vi "autonSample.vi"(0 "Auton Array":dbl[][](array[numeric]), 5 "MeasuredHeading":dbl, 9 "EncoderDistance":dbl) -> (4 "Left Drive":dbl(knob) scale=-1.0..1.0, 6 "Right Drive":dbl(knob) scale=-1.0..1.0, 10 "Misc1":dbl, 13 "Misc3":dbl, 14 "Misc4":dbl, 15 "Misc2":dbl)   [LabVIEW 2011]
uses:
  Robot Global Data.vi
  <vilib>/addons/control/pid/pid.llb/PID (DBL).vi
  <vilib>/addons/control/pid/NI_PID_pid.lvlib
panel:
  out "ArrayIndex":u16
  out "Tzero":i64
  out "AccumDist":dbl
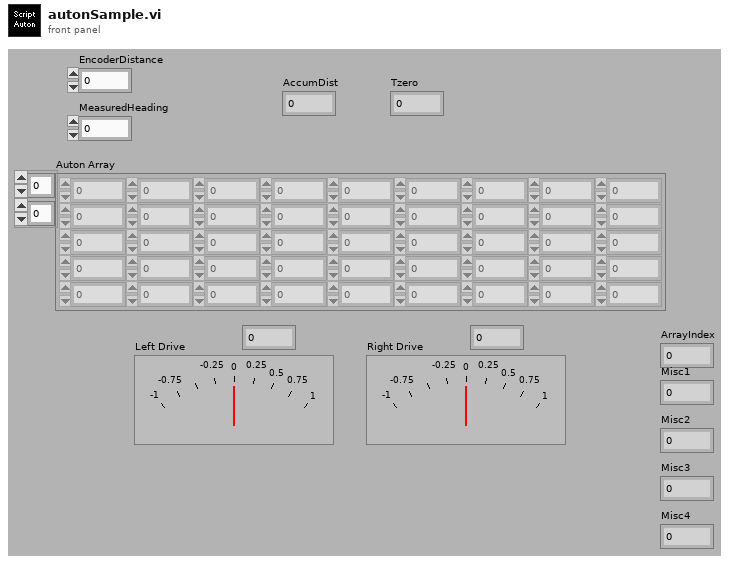
[diagram p1: front panel]
types:
  T1 = cluster{"proportional gain (Kc)":dbl, "integral time (Ti, min)":dbl, "derivative time (Td, min)":dbl}
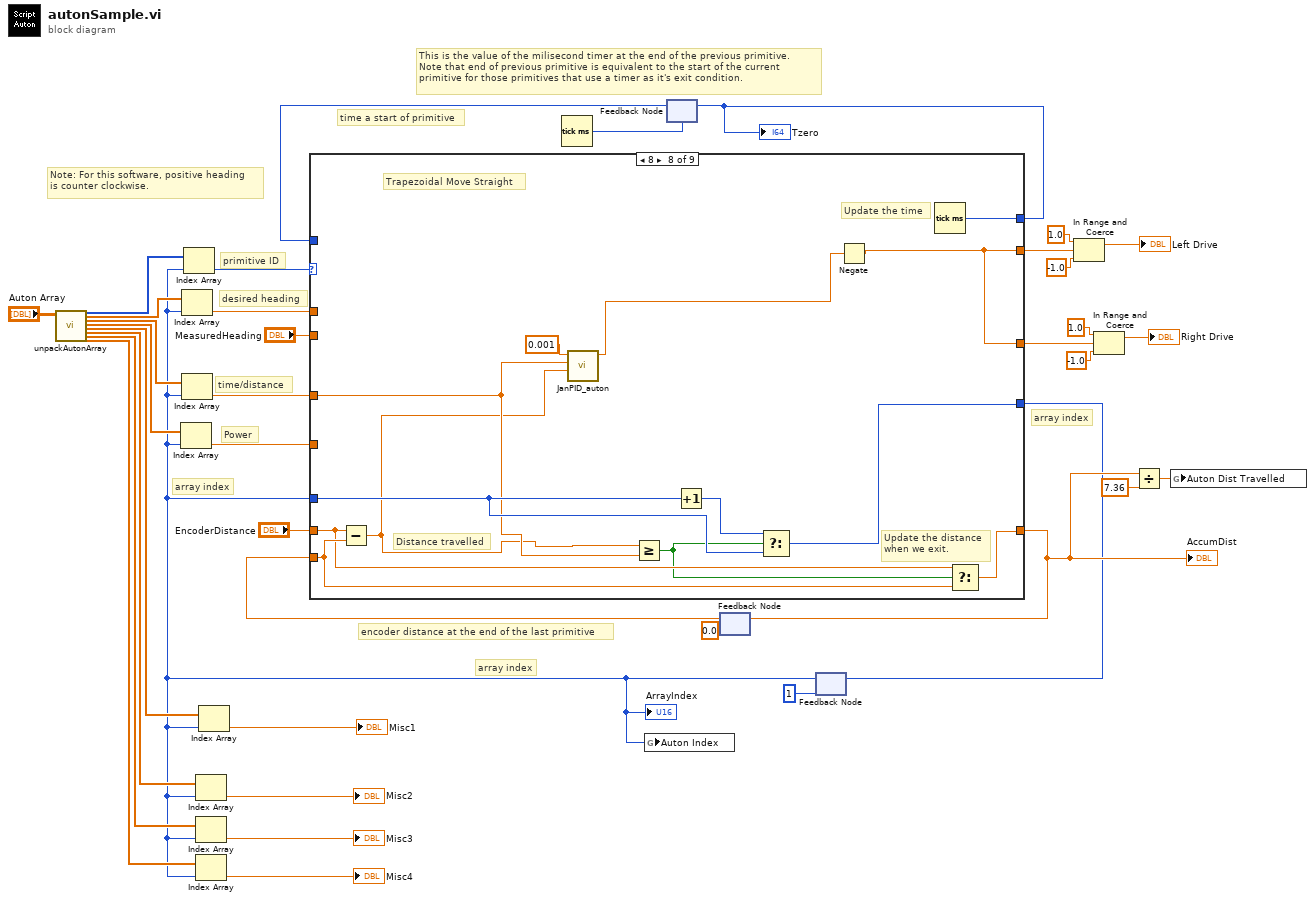
[diagram p0: block diagram]
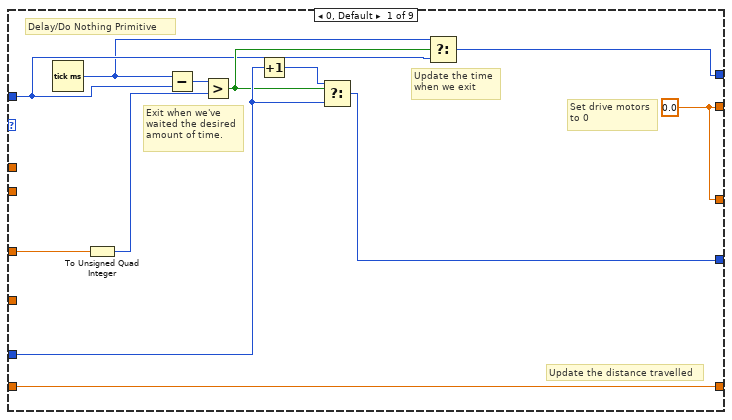
[diagram p2: hidden frame]
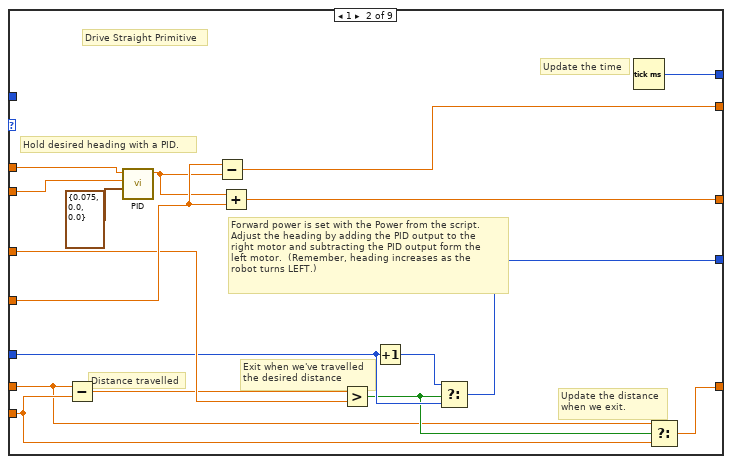
[diagram p3: hidden frame]
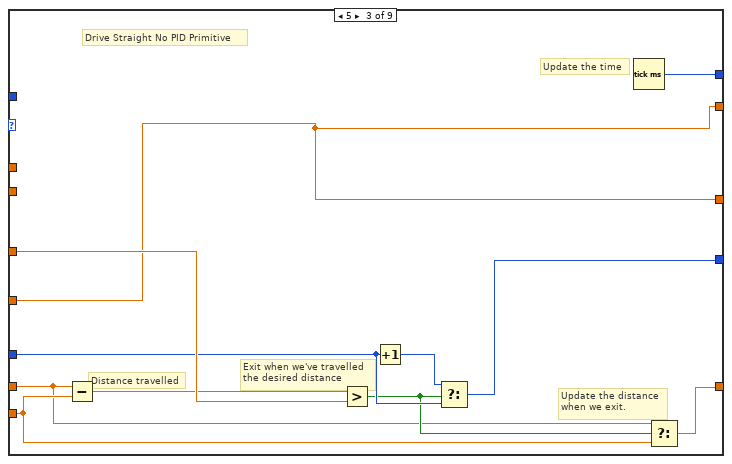
[diagram p4: hidden frame]
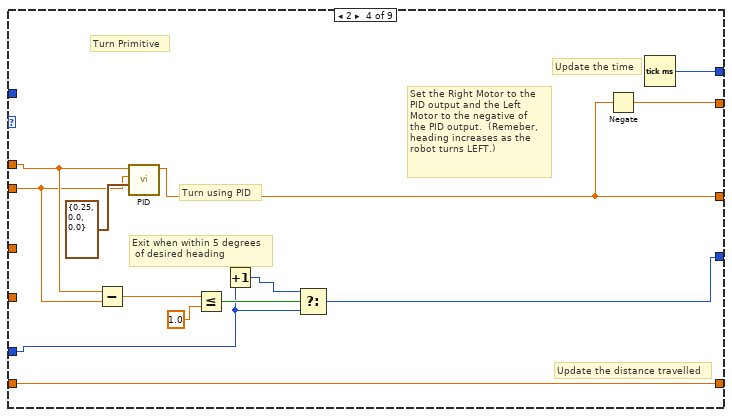
[diagram p5: hidden frame]
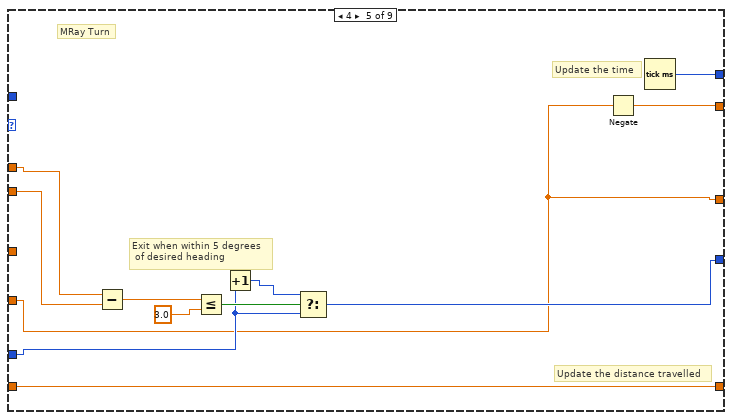
[diagram p6: hidden frame]
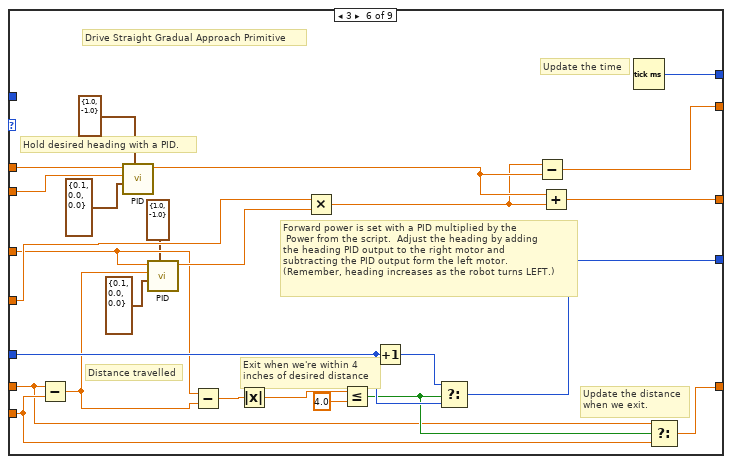
[diagram p7: hidden frame]
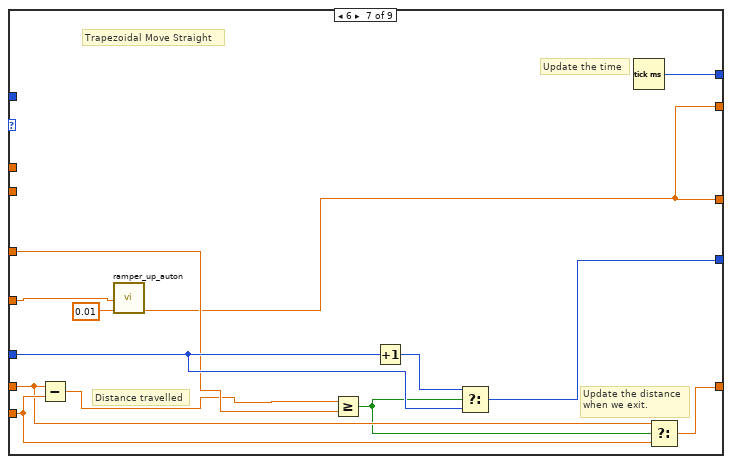
[diagram p8: hidden frame]
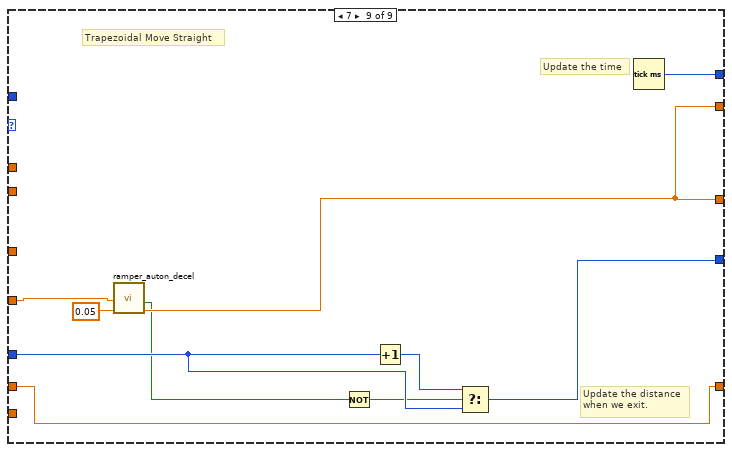
[diagram p9: hidden frame]
diagram:
  # "encoder distance at the end of the last primitive"
  # "Note: For this software, positive heading\nis counter clockwise."
  # "time a start of primitive"
  # "array index"
  # "array index"
  # "This is the value of the milisecond timer at the end of the previous primitive.\nNote that end of previous primitive is equivalent to the start of the current\nprimitive for those primitives that use a timer as it's exit condition."
  # "Power"
  # "array index"
  # "desired heading"
  # "primitive ID"
  # "time/distance"
  n1 = call "unpackAutonArray.vi"("all rows"="Auton Array") -> ("Primitive"=w37:i16[], "Heading"=w19:dbl[], "Distance/Time"=w20:dbl[], "Power"=w17:dbl[], "Misc 1"=w13:dbl[], "Misc 2"=w8:dbl[], "Misc 3"=w7:dbl[], "Misc 4"=w6:dbl[])  [unwired: 1 in, 18 out]
  n2 = Tick Count (ms)() -> (millisecond timer value=w31:u32)
  n3 = feedback #1(w31) -> (w35:u32)
  n4 = feedback #2(0.0 ("EncoderDistance")) -> (w16:dbl)
  n5 = feedback #3(1) -> (w1:i32)
  "ArrayIndex" <- w1
  n6 = Index Array(array=w17, index=w1) -> (element=w33:dbl)
  n7 = Index Array(array=w19, index=w1) -> (element=w18:dbl)
  n8 = Index Array(array=w20, index=w1) -> (element=w34:dbl)
  n9 = Index Array(array=w37, index=w1) -> (element=w36:i16)
  n10 = Index Array(array=w8, index=w1) -> (element=→"Misc2":dbl)
  n11 = Index Array(array=w7, index=w1) -> (element=→"Misc3":dbl)
  n12 = Index Array(array=w6, index=w1) -> (element=→"Misc4":dbl)
  n13 = Index Array(array=w13, index=w1) -> (element=→"Misc1":dbl)
  n14 = case shown="8" w36 {
    tunnel: [w45 w57 w75 w82 w96 w121 w139 w152 w162] -> w2
    tunnel: w1 -> [w47 w58 w76 w83 w97 w122 w140 w153 w163]
    tunnel: [w40 w56 w74 w81 w95 w120 w138 w151 w161] -> w21
    tunnel: w35 -> [w42 _ _ _ _ _ _ _ _]
    tunnel: w34 -> [w49 w60 w78 _ _ w110 w134 w146 _]
    tunnel: w18 -> [_ w67 _ w88 w102 w128 _ _ _]
    tunnel: [w44 w62 w68 w90 w103 w125 w130 w143 w158] -> w29
    tunnel: [w44 w61 w68 w89 w93 w124 w130 w143 w158] -> w22
    tunnel: w33 -> [_ w64 w68 _ w93 w112 w131 _ w159]
    tunnel: "EncoderDistance" -> [w39 w51 w69 w80 w94 w115 w135 w148 w157]
    tunnel: "MeasuredHeading" -> [_ w66 _ w87 w101 w127 _ _ _]
    tunnel: [w39 w54 w72 w80 w94 w119 w137 w150 w157] -> w4
    tunnel: w16 -> [_ w53 w71 _ _ w118 w136 w149 _]
    frame 0, Default {
      w44 = 0.0 ("Numeric")
      # "Update the distance travelled"
      # "Update the time\nwhen we exit"
      # "Exit when we've\nwaited the desired\namount of time."
      # "Set drive motors\nto 0"
      # "Delay/Do Nothing Primitive"
      n15 = Tick Count (ms)() -> (millisecond timer value=w41:u32)
      n16 = To Unsigned Quad Integer(1:w49) -> (0:w48:u64)
      n17 = Subtract(x=w41, y=w42) -> (x-y=w50:u32)
      n18 = Greater?(x=w50, y=w48) -> (0:w43:bool)
      n19 = Increment(x=w47) -> (x+1=w46:i32)
      n20 = Select(t=w46, s=w43, f=w47) -> (s? t:f=w45:i32)
      n21 = Select(t=w41, s=w43, f=w42) -> (s? t:f=w40:u32)
    }
    frame 1 {
      # "Update the distance\nwhen we exit."
      # "Distance travelled"
      # "Forward power is set with the Power from the script.\nAdjust the heading by adding the PID output to the\nright motor and subtracting the PID output form the\nleft motor.  (Remember, heading increases as the\nrobot turns LEFT.)"
      # "Hold desired heading with a PID."
      # "Update the time"
      # "Exit when we've travelled\nthe desired distance"
      # "Drive Straight Primitive"
      n22 = Subtract(x=w51, y=w53) -> (x-y=w55:dbl)
      n23 = call-poly <vilib>:"PID.vi"("PID gains"=T1 {"proportional gain (Kc)"=0.075, "integral time (Ti, min)"=0.0, "derivative time (Td, min)"=0.0}, "process variable"=w66, "setpoint"=w67) -> ("output"=w63:dbl)  [unwired: 3 in, 5 out]
      n24 = Subtract(x=w64, y=w63) -> (x-y=w62:dbl)
      n25 = Add(x=w63, y=w64) -> (x+y=w61:dbl)
      n26 = Greater?(x=w55, y=w60) -> (0:w52:bool)
      n27 = Increment(x=w58) -> (x+1=w59:i32)
      n28 = Select(t=w59, s=w52, f=w58) -> (s? t:f=w57:i32)
      n29 = Tick Count (ms)() -> (millisecond timer value=w56:u32)
      n30 = Select(t=w51, s=w52, f=w53) -> (s? t:f=w54:dbl)
    }
    frame 5 {
      # "Update the distance\nwhen we exit."
      # "Distance travelled"
      # "Update the time"
      # "Exit when we've travelled\nthe desired distance"
      # "Drive Straight No PID Primitive"
      n31 = Subtract(x=w69, y=w71) -> (x-y=w73:dbl)
      n32 = Greater?(x=w73, y=w78) -> (0:w70:bool)
      n33 = Increment(x=w76) -> (x+1=w77:i32)
      n34 = Select(t=w77, s=w70, f=w76) -> (s? t:f=w75:i32)
      n35 = Tick Count (ms)() -> (millisecond timer value=w74:u32)
      n36 = Select(t=w69, s=w70, f=w71) -> (s? t:f=w72:dbl)
    }
    frame 2 {
      # "Update the distance travelled"
      # "Set the Right Motor to the\nPID output and the Left\nMotor to the negative of\nthe PID output.  (Remeber,\nheading increases as the\nrobot turns LEFT.)"
      # "Update the time"
      # "Exit when within 5 degrees\n of desired heading"
      # "Turn using PID"
      # "Turn Primitive"
      n37 = Subtract(x=w88, y=w87) -> (x-y=w79:dbl)
      n38 = call-poly <vilib>:"PID.vi"("PID gains"=T1 {"proportional gain (Kc)"=0.25, "integral time (Ti, min)"=0.0, "derivative time (Td, min)"=0.0}, "process variable"=w87, "setpoint"=w88) -> ("output"=w89:dbl)  [unwired: 3 in, 5 out]
      n39 = Less Or Equal?(x=w79, y=1.0) -> (x <= y?=w85:bool)
      n40 = Increment(x=w83) -> (x+1=w84:i32)
      n41 = Select(t=w84, s=w85, f=w83) -> (s? t:f=w82:i32)
      n42 = Negate(x=w89) -> (-x=w90:dbl)
      n43 = Tick Count (ms)() -> (millisecond timer value=w81:u32)
    }
    frame 4 {
      # "MRay Turn"
      # "Update the distance travelled"
      # "Update the time"
      # "Exit when within 5 degrees\n of desired heading"
      n44 = Subtract(x=w102, y=w101) -> (x-y=w92:dbl)
      n45 = Less Or Equal?(x=w92, y=3.0) -> (x <= y?=w99:bool)
      n46 = Increment(x=w97) -> (x+1=w98:i32)
      n47 = Select(t=w98, s=w99, f=w97) -> (s? t:f=w96:i32)
      n48 = Negate(x=w93) -> (-x=w103:dbl)
      n49 = Tick Count (ms)() -> (millisecond timer value=w95:u32)
    }
    frame 3 {
      # "Update the distance\nwhen we exit."
      # "Distance travelled"
      # "Forward power is set with a PID multiplied by the\n Power from the script.  Adjust the heading by adding\nthe heading PID output to the right motor and \nsubtracting the PID output form the left motor.\n(Remember, heading increases as the robot turns LEFT.)"
      # "Hold desired heading with a PID."
      # "Update the time"
      # "Exit when we're within 4\ninches of desired distance"
      # "Drive Straight Gradual Approach Primitive"
      n50 = Subtract(x=w115, y=w118) -> (x-y=w108:dbl)
      n51 = call-poly <vilib>:"PID.vi"("output range"=cluster{"output high":dbl, "output low":dbl} {"output high"=1.0, "output low"=-1.0}, "PID gains"=T1 {"proportional gain (Kc)"=0.1, "integral time (Ti, min)"=0.0, "derivative time (Td, min)"=0.0}, "process variable"=w127, "setpoint"=w128) -> ("output"=w126:dbl)  [unwired: 2 in, 5 out]
      n52 = call-poly <vilib>:"PID.vi"("output range"=cluster{"output high":dbl, "output low":dbl} {"output high"=1.0, "output low"=-1.0}, "PID gains"=T1 {"proportional gain (Kc)"=0.1, "integral time (Ti, min)"=0.0, "derivative time (Td, min)"=0.0}, "process variable"=w108, "setpoint"=w110) -> ("output"=w113:dbl)  [unwired: 2 in, 5 out]
      n53 = Subtract(x=w110, y=w108) -> (x-y=w107:dbl)
      n54 = Absolute Value(x=w107) -> (abs(x)=w106:dbl)
      n55 = Multiply(x=w112, y=w113) -> (x*y=w111:dbl)
      n56 = Less Or Equal?(x=w106, y=4.0) -> (x <= y?=w117:bool)
      n57 = Increment(x=w122) -> (x+1=w123:i32)
      n58 = Select(t=w123, s=w117, f=w122) -> (s? t:f=w121:i32)
      n59 = Subtract(x=w111, y=w126) -> (x-y=w125:dbl)
      n60 = Add(x=w126, y=w111) -> (x+y=w124:dbl)
      n61 = Tick Count (ms)() -> (millisecond timer value=w120:u32)
      n62 = Select(t=w115, s=w117, f=w118) -> (s? t:f=w119:dbl)
    }
    frame 6 {
      # "Update the distance\nwhen we exit."
      # "Distance travelled"
      # "Update the time"
      # "Trapezoidal Move Straight"
      n63 = Subtract(x=w135, y=w136) -> (x-y=w133:dbl)
      n64 = call "ramper_up_auton.vi"("Rate"=0.01, "Target Setpoint"=w131) -> ("Current Setpoint"=w130:dbl)  [unwired: 9 out]
      n65 = Greater Or Equal?(x=w133, y=w134) -> (x >= y?=w129:bool)
      n66 = Increment(x=w140) -> (x+1=w141:i32)
      n67 = Select(t=w141, s=w129, f=w140) -> (s? t:f=w139:i32)
      n68 = Tick Count (ms)() -> (millisecond timer value=w138:u32)
      n69 = Select(t=w135, s=w129, f=w136) -> (s? t:f=w137:dbl)
    }
    frame 8 {
      # "Update the distance\nwhen we exit."
      # "Distance travelled"
      # "Update the time"
      # "Trapezoidal Move Straight"
      n70 = Subtract(x=w148, y=w149) -> (x-y=w145:dbl)
      n71 = call "JanPID_auton.vi"("Feedback"=w145, "Setpoint"=w146, "P"=0.001) -> ("Motor Output"=w142:dbl)  [unwired: 1 in, 7 out]
      n72 = Greater Or Equal?(x=w145, y=w146) -> (x >= y?=w147:bool)
      n73 = Increment(x=w153) -> (x+1=w154:i32)
      n74 = Select(t=w154, s=w147, f=w153) -> (s? t:f=w152:i32)
      n75 = Negate(x=w142) -> (-x=w143:dbl)
      n76 = Tick Count (ms)() -> (millisecond timer value=w151:u32)
      n77 = Select(t=w148, s=w147, f=w149) -> (s? t:f=w150:dbl)
    }
    frame 7 {
      # "Update the distance\nwhen we exit."
      # "Update the time"
      # "Trapezoidal Move Straight"
      n78 = call "ramper_auton_decel.vi"("Rate"=0.05, "Target Setpoint"=w159) -> ("Current Setpoint"=w158:dbl, "Ramping"=w155:bool)  [unwired: 8 out]
      n79 = Not(x=w155) -> (.not. x?=w156:bool)
      n80 = Increment(x=w163) -> (x+1=w164:i32)
      n81 = Select(t=w164, s=w156, f=w163) -> (s? t:f=w162:i32)
      n82 = Tick Count (ms)() -> (millisecond timer value=w161:u32)
    }
  }
  "AccumDist" <- w4
  "Tzero" <- w21
  n83 = global write "Robot Global Data.vi" "Auton Index"(w1) -> ()
  n84 = feedback-in #1(w21) -> ()
  n85 = feedback-in #2(w4) -> ()
  n86 = feedback-in #3(w2) -> ()
  n87 = In Range and Coerce(upper limit=1.0, x=w29, lower limit=-1.0) -> (coerced(x)=→"Left Drive":dbl)  [unwired: 1 out]
  n88 = In Range and Coerce(upper limit=1.0, x=w22, lower limit=-1.0) -> (coerced(x)=→"Right Drive":dbl)  [unwired: 1 out]
  n89 = Divide(x=w4, y=7.36) -> (x/y=w5:dbl)
  n90 = global write "Robot Global Data.vi" "Auton Dist Travelled"(w5) -> ()
